vi "mcapChannelLocator.get.vi"(8 "error in (no error)":errorcluster, 11 "mcap in":refnum<class "mcap.lvclass">) -> (0 "error out":errorcluster, 2 "mcapChannelLocator":refnum<class "filterTypes.lvclass">, 3 "mcap out":refnum<class "mcap.lvclass">)   [LabVIEW 2020, in "nominal types.lvlib" / "timestampManifest.lvlib" / "mcap.lvclass"]
uses:
  mcap.lvclass
  filterTypes/filterTypes.lvclass
  mcap.lvclass/mcap.ctl
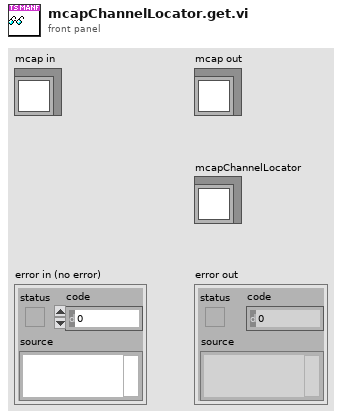
[diagram p1: front panel]
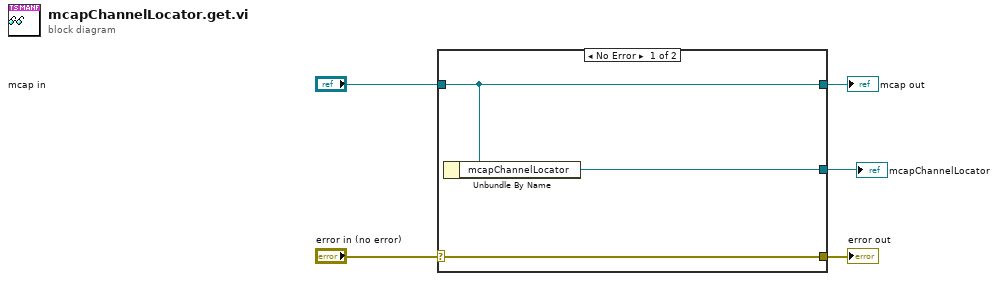
[diagram p0: block diagram]
diagram:
  n1 = case shown="No Error" "error in (no error)" {
    selector: "error in (no error)" -> [w8 w9]
    tunnel: [w8 w9] -> w4
    tunnel: [w7 w10] -> w2
    tunnel: "mcap in" -> [w7 w10]
    tunnel: [w6 _] -> w1
    frame No Error {
      n2 = Unbundle By Name(w7) -> ("mcapChannelLocator"=w6:refnum<class "filterTypes.lvclass">)
    }
    frame Error {
    }
  }
  "error out" <- w4
  "mcap out" <- w2
  "mcapChannelLocator" <- w1
